vi "Not Boolean Array (U8).vi"(4 "X":bool[](array[boolean])=[FALSE, FALSE, FALSE, FALSE, FALSE, FALSE, FALSE, TRUE]) -> (1 "Not X":bool[](array[boolean]))   [LabVIEW 2012]
doc: "This VI performs not operation on Array of Size: 8"
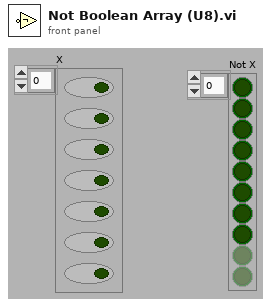
[diagram p1: front panel]
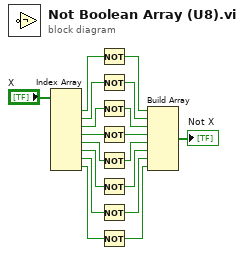
[diagram p0: block diagram]
diagram:
  n1 = Index Array(array="X") -> (element #1=w17:bool, element #2=w16:bool, element #3=w15:bool, element #4=w14:bool, element #5=w13:bool, element #6=w12:bool, element #7=w11:bool, element #8=w10:bool)  [unwired: 8 in]
  n2 = Not(x=w17) -> (.not. x?=w9:bool)
  n3 = Not(x=w16) -> (.not. x?=w8:bool)
  n4 = Not(x=w15) -> (.not. x?=w7:bool)
  n5 = Not(x=w14) -> (.not. x?=w6:bool)
  n6 = Not(x=w13) -> (.not. x?=w4:bool)
  n7 = Not(x=w12) -> (.not. x?=w5:bool)
  n8 = Not(x=w11) -> (.not. x?=w3:bool)
  n9 = Not(x=w10) -> (.not. x?=w2:bool)
  n10 = Build Array(w9, w8, w7, w6, w4, w5, w3, w2) -> (→"Not X":bool[])
